vi "Class Loader.Find Classes.vi"(8 "error in (no error)":errorcluster, 10 "base directory":path, 11 "Class Loader in":refnum<class "Class Loader.lvclass">) -> (0 "error out":errorcluster, 2 "class paths":path[](array[path]), 3 "Class Loader out":refnum<class "Class Loader.lvclass">)   [LabVIEW 2017, in "DSF.Engine.lvlib" / "Class Loader.lvclass"]
uses:
  Class Loader.lvclass
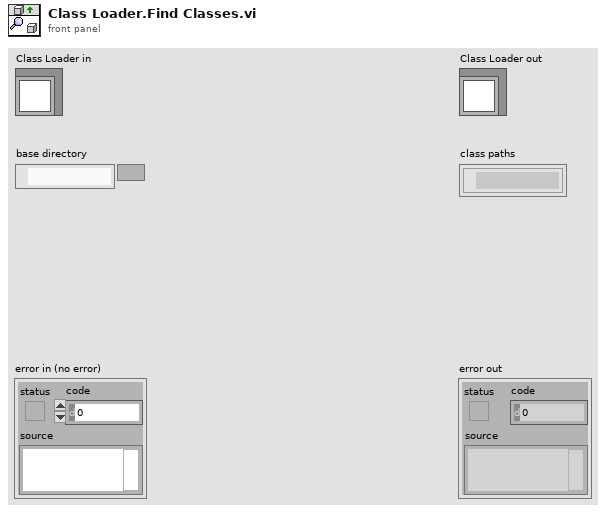
[diagram p1: front panel]
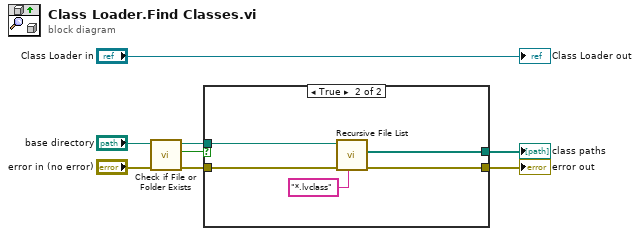
[diagram p0: block diagram]
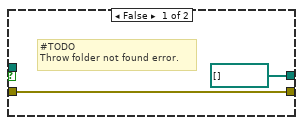
[diagram p2: hidden frame]
diagram:
  n1 = call <vilib>:"Check if File or Folder Exists.vi"("error in (no error)"="error in (no error)", "path"="base directory") -> ("error out"=w7:errorcluster, "file or folder exists?"=w8:bool, "dup path"=w6:path)  [unwired: 7 in]
  n2 = case shown="True" w8 {
    tunnel: w7 -> [w10 w13]
    tunnel: w6 -> [_ w14]
    tunnel: [w10 w12] -> w3
    tunnel: [path[] [] ("All Files in Dir") w11] -> w2
    frame False {
      # "#TODO\nThrow folder not found error."
    }
    frame True {
      n3 = call <vilib>:"Recursive File List.vi"("pattern"="*.lvclass", "error in (no error)"=w13, "Folder Path"=w14) -> ("error out"=w12:errorcluster, "All Files in Dir"=w11:path[])  [unwired: 4 in, 3 out]
    }
  }
  "error out" <- w3
  "class paths" <- w2
  "Class Loader out" <- "Class Loader in"
